vi "02-01-17.vi"() -> ()   [LabVIEW 2016]
panel:
  out "XY Graph 5":cluster{dbl[], dbl[]}[](graph)
  out "XY Graph 4":cluster{dbl[], dbl[]}[](graph)
  out "XY Graph 3":cluster{dbl[], dbl[]}[](graph)
  out "XY Graph 2":cluster{dbl[], dbl[]}[](graph)
  out "XY Graph":cluster{dbl[], dbl[]}[](graph)
  # "2x Coulson @3700-3750 RPM"
  # "Drive signal window @ +-75"
  # "@+-50"
  # "@+-25 (--> +-50)"
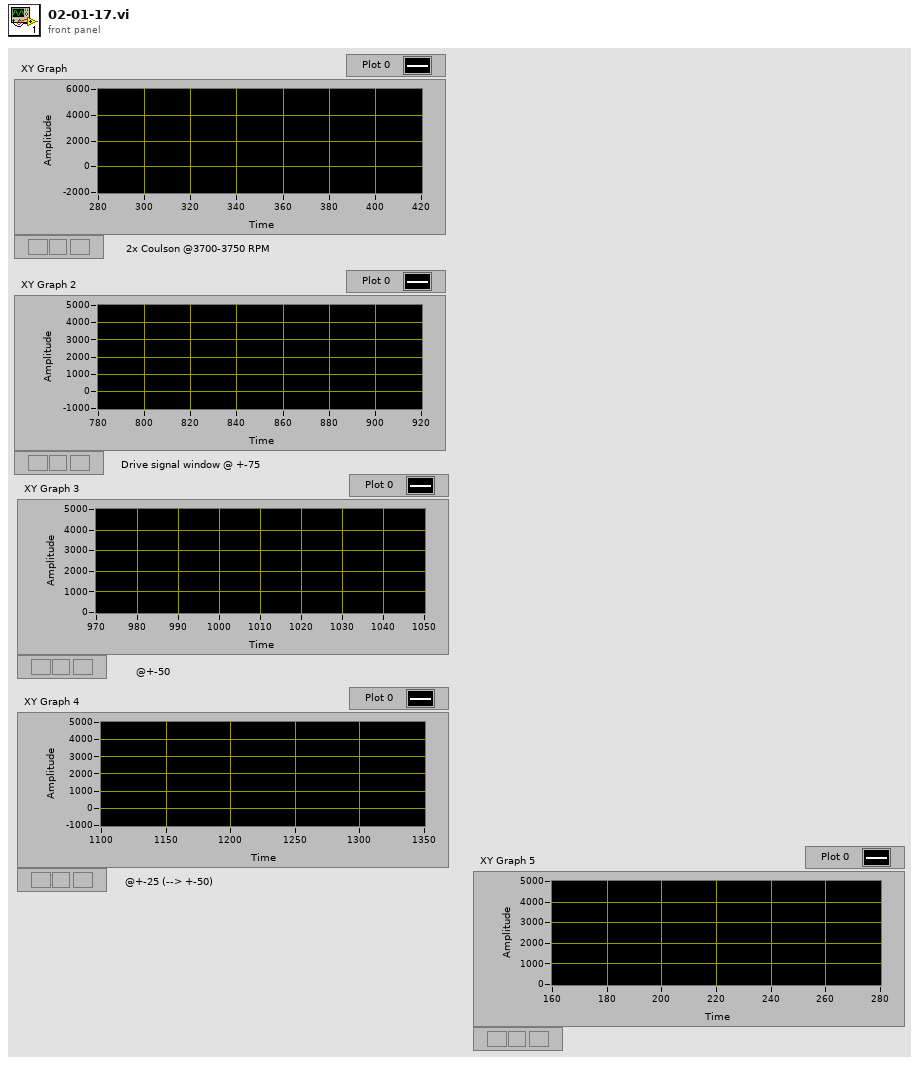
[diagram p1: front panel]
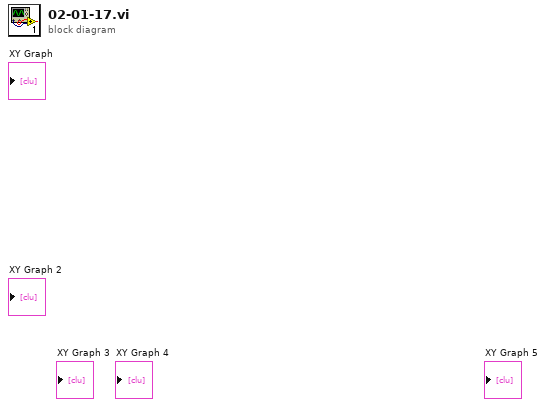
[diagram p0: block diagram]
diagram:
